vi "GPS correct.vi"(1 "Raw Longitude":dbl) -> (0 "Corrected Longitude":dbl)   [LabVIEW 2009]
panel:
  # "This correction value system only works for\nlongituted between 42-43.5 degrees."
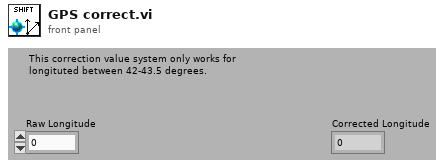
[diagram p1: front panel]
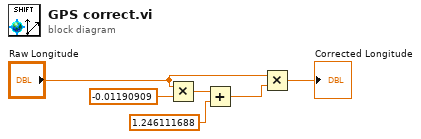
[diagram p0: block diagram]
diagram:
  n1 = Multiply(x="Raw Longitude", y=-0.01190909) -> (x*y=w5:dbl)
  n2 = Add(x=w5, y=1.246111688) -> (x+y=w2:dbl)
  n3 = Multiply(x="Raw Longitude", y=w2) -> (x*y=→"Corrected Longitude":dbl)
